vi "Write Instr.vi"(8 "error in (no error)":errorcluster, 10 "Instrument.lvclass":refnum<class "Instrument.lvclass">, 11 "Instr Actor in":refnum<class "Instr Actor.lvclass">) -> (0 "error out":errorcluster, 3 "Instr Actor out":refnum<class "Instr Actor.lvclass">)   [LabVIEW 2014, in "Instrument Library.lvlib" / "Instr Actor.lvclass"]
uses:
  Instr Actor.lvclass
  reusable/Instrument/Instrument.lvclass
  Instr Actor.lvclass/Instr Actor.ctl
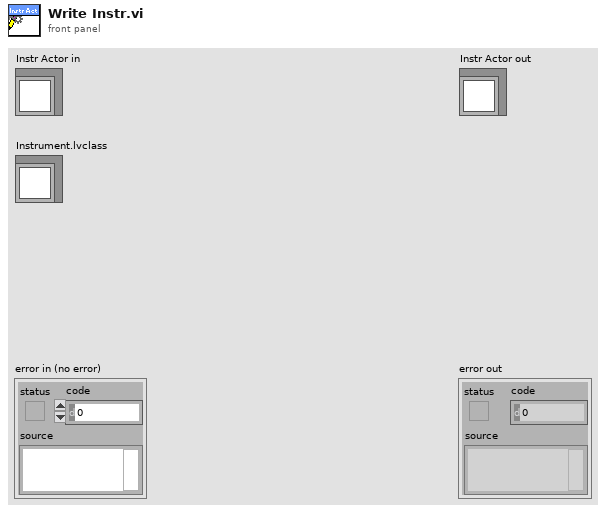
[diagram p1: front panel]
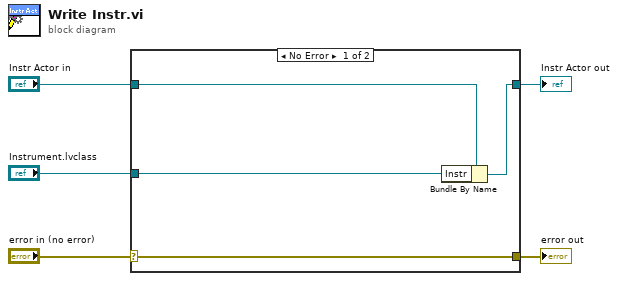
[diagram p0: block diagram]
diagram:
  n1 = case shown="No Error" "error in (no error)" {
    selector: "error in (no error)" -> [w9 w10]
    tunnel: [w9 w10] -> w4
    tunnel: [w7 w11] -> w2
    tunnel: "Instr Actor in" -> [w8 w11]
    tunnel: "Instrument.lvclass" -> [w6 _]
    frame No Error {
      n2 = Bundle By Name(cluster=w8, "Instr"=w6) -> (w7:refnum<class "Instr Actor.lvclass">)
    }
    frame Error {
    }
  }
  "error out" <- w4
  "Instr Actor out" <- w2
